vi "MoveMI_in_lat.vi"(8 "error in (no error)":errorcluster) -> (0 "error out":errorcluster, 3 "No errors =T":bool)   [LabVIEW 2020]
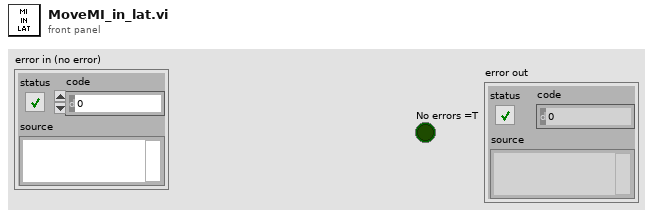
[diagram p1: front panel]
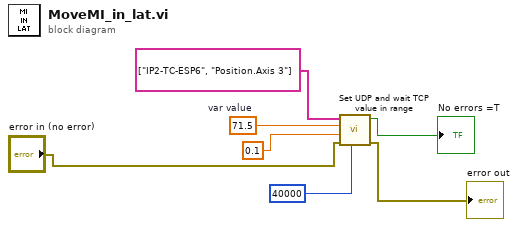
[diagram p0: block diagram]
diagram:
  w7 = 71.5  # var value
  n1 = call "Set UDP and wait TCP value in range.vi"("timeout"=40000 ("slow timeout ms (3000)"), "error in (no error)"="error in (no error)", "tolerance"=0.1, "set value"=w7, "device and variable"=string[] ["IP2-TC-ESP6", "Position.Axis 3"] ("dev variable alias Motors X")) -> ("error out"=→"error out":errorcluster, "In range is True"=→"No errors =T":bool)  [unwired: 5 in]
